vi "DMM Configuration - Get RTD-Thermistor ABC Param.vi"(8 "error in (no error)":errorcluster, 11 "DMM Temp - Value In":T1={"DMM Temp - Transducer Type"=1, "DMM Temp - Thermocouple Type"=6, "DMM Temp - Fixed Reference Junction"=25.0, "DMM Temp - RTD Type"=enum."Pt3851", "DMM Temp - RTD Resistance"=100.0, "DMM Temp - Thermistor Type"=enum."44006", "DMM Temp - RTD A"=0.0039083, "DMM Temp - RTD B"=-5.775e-07, "DMM Temp - RTD C"=-4.183e-12, "DMM Temp - Thermistor A"=0.0010295, "DMM Temp - Thermistor B"=0.0002391, "DMM Temp - Thermistor C"=1.568e-07} {"DMM Temp - Thermistor C" format="%#_13g"; "DMM Temp - Thermistor B" format="%#_13g"; "DMM Temp - Thermistor A" format="%#_13g"; "DMM Temp - RTD Resistance" format="%.2f"; "DMM Temp - Fixed Reference Junction" format="%.2f"; "DMM Temp - Thermocouple Type" items=["B"=1, "E"=4, "J"=6, "K"=7, "N"=8, "R"=9, "S"=10, "T"=11]; "DMM Temp - Transducer Type" items=["Thermocouple"=1, "Thermistor"=2, "2-Wire RTD"=3, "4-Wire RTD"=4]}) -> (0 "error out":errorcluster, 3 "DMM Temp - Value Out":T1={"DMM Temp - Transducer Type"=1, "DMM Temp - Thermocouple Type"=6, "DMM Temp - Fixed Reference Junction"=25.0, "DMM Temp - RTD Type"=enum."Pt3851", "DMM Temp - RTD Resistance"=100.0, "DMM Temp - Thermistor Type"=enum."44006", "DMM Temp - RTD A"=0.0039083, "DMM Temp - RTD B"=-5.775e-07, "DMM Temp - RTD C"=-4.183e-12, "DMM Temp - Thermistor A"=0.0010295, "DMM Temp - Thermistor B"=0.0002391, "DMM Temp - Thermistor C"=1.568e-07} {"DMM Temp - Thermistor C" format="%#_13g"; "DMM Temp - Thermistor B" format="%#_13g"; "DMM Temp - Thermistor A" format="%#_13g"; "DMM Temp - RTD Resistance" format="%.2f"; "DMM Temp - Fixed Reference Junction" format="%.2f"; "DMM Temp - Thermocouple Type" items=["B"=1, "E"=4, "J"=6, "K"=7, "N"=8, "R"=9, "S"=10, "T"=11]; "DMM Temp - Transducer Type" items=["Thermocouple"=1, "Thermistor"=2, "2-Wire RTD"=3, "4-Wire RTD"=4]})   [LabVIEW 2016, in "DMM-SWITCH-ScanList System Explorer.lvlib"]
uses:
  DMM-SWITCH-ScanList System Explorer.lvlib
  Configuration Controls/DMM Temp.ctl
  <instrlib>/niDMM/nidmm.llb/niDMM Transducer Type.ctl
  <instrlib>/niDMM/nidmm.llb/niDMM Thermocouple Type.ctl
  <instrlib>/niDMM/nidmm.llb/niDMM RTD Type.ctl
  <instrlib>/niDMM/nidmm.llb/niDMM Thermistor Type.ctl
panel:
  in  "OK":bool
  in  "C":dbl
  in  "B":dbl
  in  "A":dbl
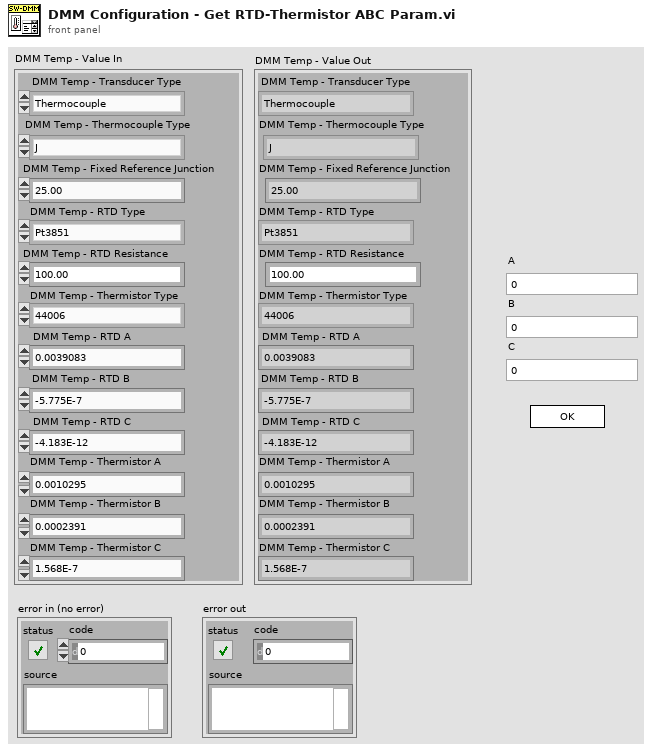
[diagram p1: front panel]
types:
  T1 = typedef "DMM-SWITCH-ScanList System Explorer.lvlib/DMM Temp.ctl" = cluster{"DMM Temp - Transducer Type":T2, "DMM Temp - Thermocouple Type":T3, "DMM Temp - Fixed Reference Junction":dbl, "DMM Temp - RTD Type":T4, "DMM Temp - RTD Resistance":dbl, "DMM Temp - Thermistor Type":T5, "DMM Temp - RTD A":dbl, "DMM Temp - RTD B":dbl, "DMM Temp - RTD C":dbl, "DMM Temp - Thermistor A":dbl, "DMM Temp - Thermistor B":dbl, "DMM Temp - Thermistor C":dbl}
  T2 = typedef "niDMM Transducer Type.ctl" = i32
  T3 = typedef "niDMM Thermocouple Type.ctl" = i32
  T4 = typedef "niDMM RTD Type.ctl" = enum16{"Custom", "Pt3750", "Pt3851", "Pt3911", "Pt3916", "Pt3920", "Pt3928"}
  T5 = typedef "niDMM Thermistor Type.ctl" = enum16{"Custom", "44004", "44006", "44007"}
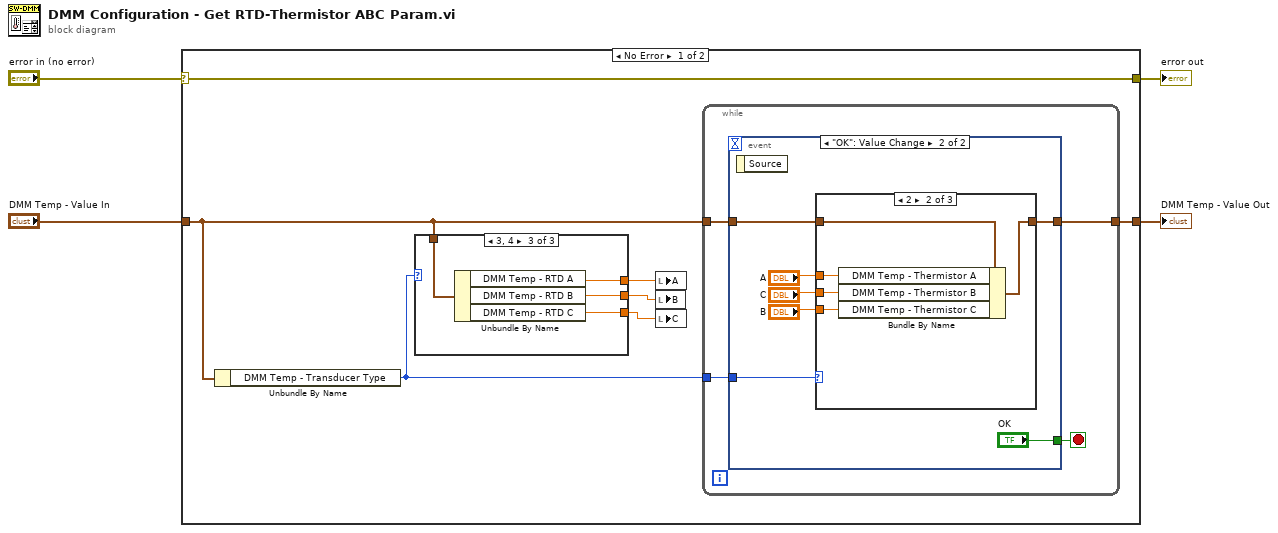
[diagram p0: block diagram]
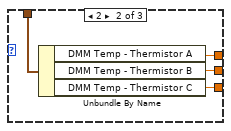
[diagram p3: hidden frame]
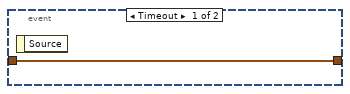
[diagram p4: hidden frame]
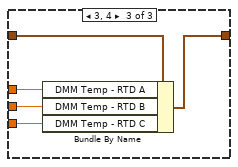
[diagram p6: hidden frame]
diagram:
  n1 = case shown="No Error" "error in (no error)" {
    selector: "error in (no error)" -> [w5 w44]
    tunnel: [w11 w43] -> w4
    tunnel: "DMM Temp - Value In" -> [w7 w43]
    tunnel: [w5 w44] -> w1
    frame No Error {
      n2 = Unbundle By Name(w7) -> ("DMM Temp - Transducer Type"=w6:T2)
      n3 = case shown="3, 4" w6 {
        tunnel: w7 -> [_ w15 w19]
        tunnel: [_ w14 w18] -> w10
        tunnel: [_ w13 w17] -> w9
        tunnel: [_ w12 w16] -> w8
        frame 0, Default {
        }
        frame 2 {
          n4 = Unbundle By Name(w15) -> ("DMM Temp - Thermistor A"=w12:dbl, "DMM Temp - Thermistor B"=w13:dbl, "DMM Temp - Thermistor C"=w14:dbl)
        }
        frame 3, 4 {
          n5 = Unbundle By Name(w19) -> ("DMM Temp - RTD A"=w16:dbl, "DMM Temp - RTD B"=w17:dbl, "DMM Temp - RTD C"=w18:dbl)
        }
      }
      n6 = local write "A"(w8) -> ()
      n7 = local write "B"(w9) -> ()
      n8 = local write "C"(w10) -> ()
      n9 = while {
        tunnel: w7 -> [w22]
        tunnel: [w21] -> w11
        tunnel: w6 -> [w20]
        stop <- w23 stop-if-true
        n10 = event shown="[1] \"OK\": Value Change" {
          selector: _ -> [_ _]
          dyn-events: _ -> [_ _]
          timeout: _ -> [_ _]
          tunnel: [_ "OK"] -> w23
          tunnel: w22 -> [w24 w30]
          tunnel: [w24 w26] -> w21
          tunnel: w20 -> [_ w25]
          event Timeout {
            n11 = event-data() -> ()  [unwired: 1 in, 1 out]
          }
          event "OK": Value Change {
            n12 = event-data() -> ()  [unwired: 1 in, 1 out]
            n13 = case shown="2" w25 {
              tunnel: w30 -> [w32 w37 w42]
              tunnel: "A" -> [_ w36 w41]
              tunnel: "C" -> [_ w35 w40]
              tunnel: "B" -> [_ w34 w39]
              tunnel: [w32 w33 w38] -> w26
              frame 0, Default {
              }
              frame 2 {
                n14 = Bundle By Name(cluster=w37, "DMM Temp - Thermistor A"=w36, "DMM Temp - Thermistor B"=w35, "DMM Temp - Thermistor C"=w34) -> (w33:T1)
              }
              frame 3, 4 {
                n15 = Bundle By Name(cluster=w42, "DMM Temp - RTD A"=w41, "DMM Temp - RTD B"=w40, "DMM Temp - RTD C"=w39) -> (w38:T1)
              }
            }
          }
        }
      }
    }
    frame Error {
    }
  }
  "error out" <- w1
  "DMM Temp - Value Out" <- w4
